vi "Make Label Line.vi"(1 "Column Names":string[](array[string]), 2 "File Name":string="Test.001") -> (0 "Igor Column Headings":string)   [LabVIEW 2024]
doc: "This VI takes an input array of column names and outputs a single string of appropriately spaced column names in a format that Igor will accept for automatically nameing the columns. The file index number is appended to each column name to keep sequential data files separate\nScott Hannahs, NHMFL-FSU, February 1995"
uses:
  <vilib>/Utility/error.llb/Trim Whitespace One-Sided.vi
  <vilib>/regexp/Match Regular Expression.xnode
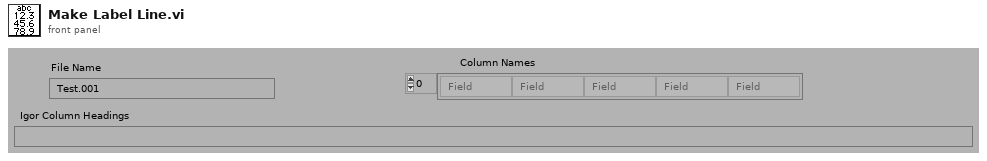
[diagram p1: front panel]
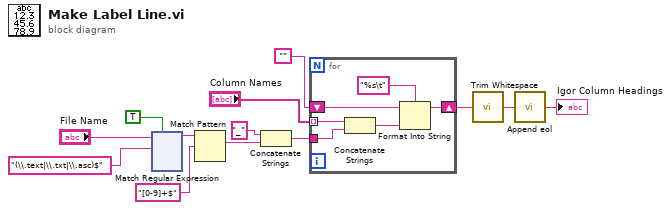
[diagram p0: block diagram]
diagram:
  n1 = xnode "Match Regular Expression"("input string"="File Name", "regular expression"="(\\.text|\\.txt|\\.asc)$", "ignore case? (F)"=TRUE) -> ("before match"=w4:string)  [unwired: 3 in, 4 out]
  n2 = Match Pattern(string=w4, regular expression="[0-9]+$") -> (match substring=w8:string)  [unwired: 1 in, 3 out]
  n3 = Concatenate Strings("_", w8) -> (w7:string)
  n4 = for {
    tunnel: "Column Names" -> [w19] mode=indexing
    shift-right: [w14] -> w12
    shift-left: "" -> [w15]
    tunnel: w7 -> [w18]
    n5 = Concatenate Strings(w19, w18) -> (w16:string)
    n6 = Format Into String(format string="%s\t", initial string=w15, w16) -> (resulting string=w14:string)  [unwired: 1 in, 1 out]
  }
  n7 = call <vilib>:"Trim Whitespace.vi"("string"=w12) -> ("trimmed string"=w5:string)  [unwired: 1 in]
  n8 = call "Append eol.vi"("INPUT STRING"=w5) -> ("OUTPUT STRING (PLUS End of Line)"=→"Igor Column Headings":string)
